vi "ExportExcelValues.vi"(8 "error in (no error)":errorcluster, 9 "Contents":string[][](array[string]), 10 "Current Title":string[](array[string])=["PCB标识", "封装", "规格", "型号", "品牌", "单板数量", "备注"], 11 "Excel in":refnum<class "Excel.lvclass">) -> (0 "error out":errorcluster, 3 "Excel out":refnum<class "Excel.lvclass">)   [LabVIEW 2015, in "Excel.lvclass"]
uses:
  Excel.lvclass
  <vilib>/addons/_office/_exclsub.llb/font.ctl
  <vilib>/addons/_office/excel.llb/Excel Easy Table (str).vi
  <vilib>/addons/_office/NI_ReportGenerationToolkit.lvlib
  <vilib>/Utility/NIReport.llb/NI_report.lvclass
  <vilib>/Utility/NIReport.llb/Excel/NI_Excel.lvclass
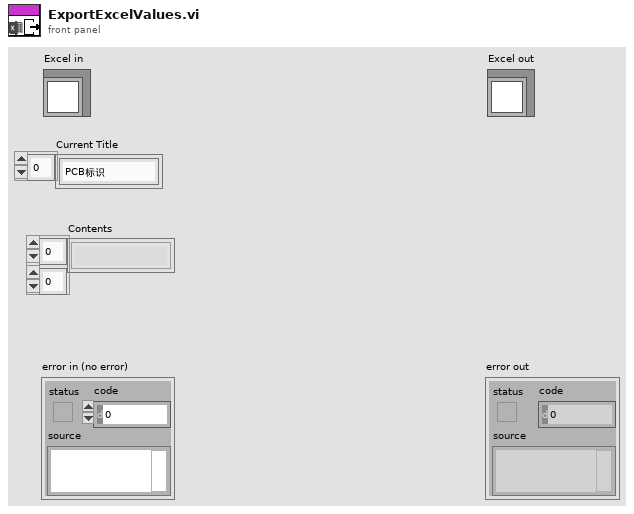
[diagram p1: front panel]
types:
  T1 = typedef "NI_ReportGenerationToolkit.lvlib/font.ctl" = cluster{"font name":string, "font size":dbl, "bold":u16, "italic":u16, "underline":u16, "strike through":u16, "font color":u32}
  T2 = enum16{"maximized", "minimized", "normal", "no change"}
  T3 = enum16{"Standard Report", "HTML", "Word", "Excel"}
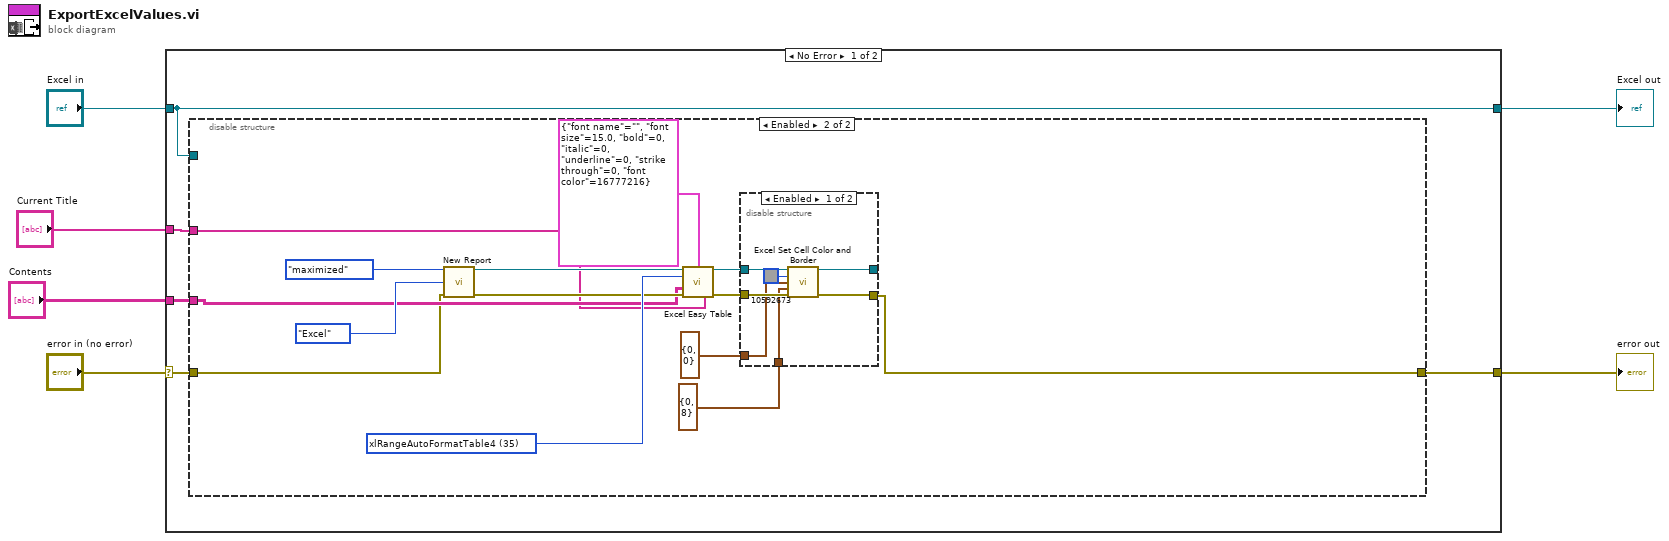
[diagram p0: block diagram]
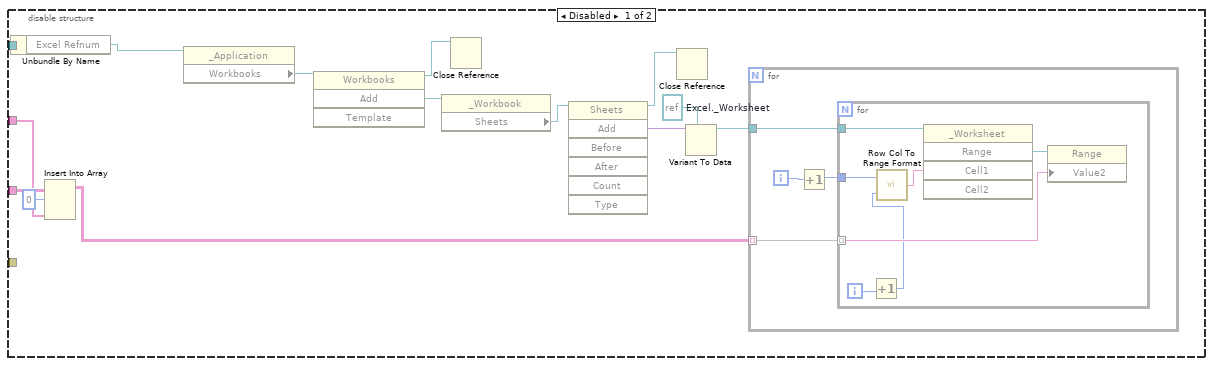
[diagram p2: hidden frame]
diagram:
  n1 = case shown="No Error" "error in (no error)" {
    selector: "error in (no error)" -> [w8 w59]
    tunnel: [w7 w59] -> w5
    tunnel: [w11 w58] -> w4
    tunnel: "Excel in" -> [w11 w58]
    tunnel: "Current Title" -> [w9 _]
    tunnel: "Contents" -> [w10 _]
    frame No Error {
      n2 = disable-structure shown="Enabled" {
        disable-tunnel: w11 -> [w18 _]
        disable-tunnel: w10 -> [w16 w41]
        disable-tunnel: w9 -> [w14 w40]
        disable-tunnel: w8 -> [_ w39]
        disable-tunnel: [_ w38] -> w7
        frame Disabled {
          w19 = refnum<k7> refnum  # Excel._Worksheet
          n3 = Unbundle By Name(w18) -> ("Excel Refnum"=w17:refnum<k7>)
          n4 = Insert Into Array(array=w16, index (row)=0, new element=w14) -> (w13:string[][])  [unwired: 1 in]
          n5 = property class="_Application"(reference=w17) -> ("Workbooks"=w25:refnum<k7>)  [unwired: 1 in, 2 out]
          n6 = invoke class="Workbooks" method="Add"(reference=w25) -> (reference out=w24:refnum<k7>, "Add"=w23:refnum<k7>)  [unwired: 3 in, 2 out]
          n7 = property class="_Workbook"(reference=w23) -> ("Sheets"=w22:refnum<k7>)  [unwired: 1 in, 2 out]
          n8 = Close Reference(reference=w24) -> ()  [unwired: 1 in, 1 out]
          n9 = invoke class="Sheets" method="Add"(reference=w22) -> (reference out=w21:refnum<k7>, "Add"=w20:variant)  [unwired: 6 in, 5 out]
          n10 = Close Reference(reference=w21) -> ()  [unwired: 1 in, 1 out]
          n11 = Variant To Data(type=w19, Variant=w20) -> (data=w12:refnum<k7>)  [unwired: 1 in, 1 out]
          n12 = for {
            tunnel: w13 -> [w28] mode=indexing
            tunnel: w12 -> [w29]
            i -> [w27]
            n13 = Increment(x=w27) -> (x+1=w26:i32)
            n14 = for {
              tunnel: w26 -> [w36]
              tunnel: w29 -> [w35]
              tunnel: w28 -> [w32] mode=indexing
              i -> [w31]
              n15 = Increment(x=w31) -> (x+1=w30:i32)
              n16 = call "Row Col To Range Format.vi"("Column"=w30, "Row"=w36) -> ("Output String"=w34:string)
              n17 = invoke class="_Worksheet" method="Range"(reference=w35, "Cell1"=w34) -> ("Range"=w33:refnum<k7>)  [unwired: 3 in, 4 out]
              n18 = property class="Range"(reference=w33, "Value2"=w32) -> ()  [unwired: 1 in, 2 out]
            }
          }
        }
        frame Enabled {
          w48 = 35 items=["xlRangeAutoFormat3DEffects1"=13, "xlRangeAutoFormat3DEffects2"=14, "xlRangeAutoFormatAccounting1"=4, "xlRangeAutoFormatAccounting2"=5, "xlRangeAutoFormatAccounting3"=6, "xlRangeAutoFormatAccounting4"=17, "xlRangeAutoFormatClassic1"=1, "xlRangeAutoFormatClassic2"=2, "xlRangeAutoFormatClassic3"=3, "xlRangeAutoFormatColor1"=7, "xlRangeAutoFormatColor2"=8, "xlRangeAutoFormatColor3"=9, "xlRangeAutoFormatList1"=10, "xlRangeAutoFormatList2"=11, "xlRangeAutoFormatList3"=12, "xlRangeAutoFormatLocalFormat1"=15, "xlRangeAutoFormatLocalFormat2"=16, "xlRangeAutoFormatLocalFormat3"=19, "xlRangeAutoFormatLocalFormat4"=20, "xlRangeAutoFormatReport1"=21, "xlRangeAutoFormatReport2"=22, "xlRangeAutoFormatReport3"=23, "xlRangeAutoFormatReport4"=24, "xlRangeAutoFormatReport5"=25, "xlRangeAutoFormatReport6"=26, "xlRangeAutoFormatReport7"=27, "xlRangeAutoFormatReport8"=28, "xlRangeAutoFormatReport9"=29, "xlRangeAutoFormatReport10"=30, "xlRangeAutoFormatClassicPivotTable"=31, "xlRangeAutoFormatTable1"=32, "xlRangeAutoFormatTable2"=33, "xlRangeAutoFormatTable3"=34, "xlRangeAutoFormatTable4"=35, "xlRangeAutoFormatTable5"=36, "xlRangeAutoFormatTable6"=37, "xlRangeAutoFormatTable7"=38, "xlRangeAutoFormatTable8"=39, "xlRangeAutoFormatTable9"=40, "xlRangeAutoFormatTable10"=41, "xlRangeAutoFormatPTNone"=42, "xlRangeAutoFormatNone"=-4142, "xlRangeAutoFormatSimple"=-4154] ("auto format (none)")
          n19 = call <vilib>:"New Report.vi"("window state (normal)"=T2."maximized", "report type"=T3."Excel", "error in (no error)"=w39) -> ("report out"=w43:refnum<class "NI_report.lvclass">, "error out"=w42:errorcluster)  [unwired: 11 in]
          n20 = call-poly <vilib>:"Excel Easy Table.vi"("report in"=w43, "font"=T1 {"font name"="", "font size"=15.0, "bold"=0, "italic"=0, "underline"=0, "strike through"=0, "font color"=16777216}, "auto format (none)"=w48, "text data"=w41, "error in (no error)"=w42, "column headers"=w40) -> ("report out"=w47:refnum<class "NI_report.lvclass">, "error out"=w46:errorcluster)  [unwired: 5 in, 3 out]
          n21 = disable-structure shown="Enabled" {
            disable-tunnel: w47 -> [w57 _]
            disable-tunnel: w46 -> [w56 _]
            disable-tunnel: cluster{"row":i32, "column":i32} {"row"=0, "column"=0} ("start (-1, -1)") -> [w54 _]
            disable-tunnel: cluster{"row":i32, "column":i32} {"row"=0, "column"=8} ("end (-1, -1)") -> [w53 _]
            disable-tunnel: [w52 _] -> _
            disable-tunnel: [w51 _] -> w38
            frame Enabled {
              n22 = call <vilib>:"Excel Set Cell Color and Border.vi"("report in"=w57, "background color (w)"=u32 10592673, "start (-1, -1)"=w54, "end (-1, -1)"=w53, "error in (no error)"=w56) -> ("report out"=w52:refnum<class "NI_report.lvclass">, "error out"=w51:errorcluster)  [unwired: 9 in]
            }
            frame Disabled {
            }
          }
        }
      }
    }
    frame Error {
    }
  }
  "error out" <- w5
  "Excel out" <- w4
